vi "GetPrivateNotifierStatus.vi"(8 "error in (no error)":errorcluster, 11 "DAQmx":refnum<class "DAQmx.lvclass">) -> (0 "error out":errorcluster, 2 "State":T1, 3 "DAQmx out":refnum<class "DAQmx.lvclass">)   [LabVIEW 2019, in "DAQmx.lvclass"]
uses:
  DAQmx.lvclass
  typedefs/DAQmx.States--enum.ctl
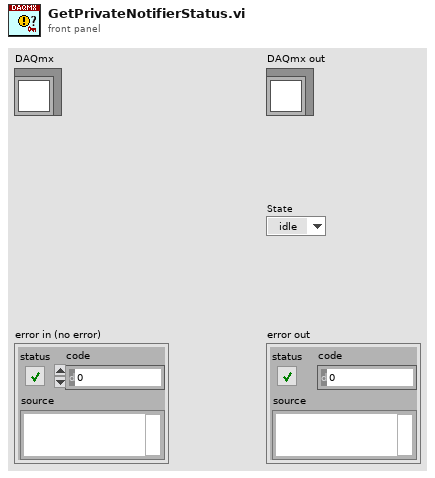
[diagram p1: front panel]
types:
  T1 = typedef "DAQmx.lvclass/DAQmx.States--enum.ctl" = enum16{"idle", "start", "stop", "calibrate", "auto", "exit"}
  T2 = typedef "DAQmx.lvclass/DAQ.Config.Timing--Cluster.ctl" = cluster{"Sampling":T3, "sample mode":i32, "FsMode":T4, "Fs Multiplier":dbl, "Refresh Rate (Hz)":dbl, "Decimation.PreDSP":i32, "Decimation.PostDSP":i32, "Fs.Output":dbl}
  T3 = typedef "DAQmx.lvclass/DAQ.Config.Timing.Sampling--Cluster.ctl" = cluster{"Fs":dbl, "#s":i32}
  T4 = typedef "DAQmx.lvclass/DAQ.Config.Timing.Fs Mode--enum.ctl" = enum16{"Manual", "Auto Fs", "Max Fs"}
  T5 = typedef "DAQmx.lvclass/DAQ.Config.AI--Cluster--Array.ctl" = T6[]
  T6 = typedef "DAQmx.lvclass/DAQ.Config.AI--Cluster.ctl" = cluster{"Channels":tag, "Coupling":T7, "Range":T8, "input terminal configuration":i32, "Type":T9}
  T7 = typedef "DAQmx.lvclass/DAQ.Config.AI.Coupling--enum.ctl" = u16
  T8 = typedef "DAQmx.lvclass/DAQ.Config.AI.Range--enum.ctl" = enum16{"±0.316", "±1.00", "±3.16", "±10.0", "±31.6", "±42.4", ""}
  T9 = typedef "DAQmx.lvclass/DAQ.Config.Device Type--enum.ctl" = enum16{"None", "USB-4431", "PXI-446x"}
  T10 = typedef "DAQmx.lvclass/DAQ.Config.AO--Cluster--Array.ctl" = T11[]
  T11 = typedef "DAQmx.lvclass/DAQ.Config.AO--Cluster.ctl" = cluster{"Channels":tag, "Range":T12, "output terminal configuration":i32, "Type":T9}
  T12 = typedef "DAQmx.lvclass/DAQ.Config.AO.Range--enum.ctl" = enum16{"±0.1", "±1.0", "±10.0", ""}
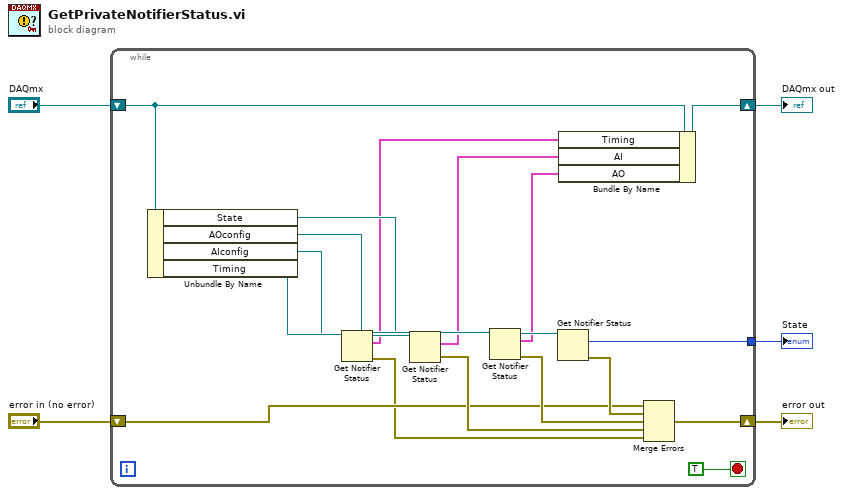
[diagram p0: block diagram]
diagram:
  n1 = while {
    shift-right: [w6] -> w4
    shift-left: "DAQmx" -> [w8]
    shift-right: [w10] -> w2
    shift-left: "error in (no error)" -> [w12]
    tunnel: [w7] -> w1
    stop <- TRUE stop-if-true
    n2 = Unbundle By Name(w8) -> ("State"=w19:refnum<user-event>, "AOconfig"=w20:refnum<user-event>, "AIconfig"=w21:refnum<user-event>, "Timing"=w22:refnum<user-event>)
    n3 = Get Notifier Status(notifier=w22) -> (current notification=w16:T2, error out=w11:errorcluster)  [unwired: 1 in, 3 out]
    n4 = Get Notifier Status(notifier=w21) -> (current notification=w17:T5, error out=w13:errorcluster)  [unwired: 1 in, 3 out]
    n5 = Get Notifier Status(notifier=w20) -> (current notification=w18:T10, error out=w14:errorcluster)  [unwired: 1 in, 3 out]
    n6 = Get Notifier Status(notifier=w19) -> (current notification=w7:T1, error out=w15:errorcluster)  [unwired: 1 in, 3 out]
    n7 = Bundle By Name(cluster=w8, "Timing"=w16, "AI"=w17, "AO"=w18) -> (w6:refnum<class "DAQmx.lvclass">)
    n8 = Merge Errors(w12, w15, w14, w13, w11) -> (w10:errorcluster)
  }
  "error out" <- w2
  "DAQmx out" <- w4
  "State" <- w1
